vi "3D_send_CCS_command.vi"(0 "CCS IP":string="192.168.000.002", 1 "Intensity 0-255":u8=255, 2 "Light mode":T1(ring), 3 "On/off":bool, 5 "remote port or service name":u16=40001, 7 "Select CCS channel":u16(ring)=2 items=["Chanel 00", "Chanel 01", "Chanel 02"], 9 "Select CCS property":u16(ring)=2 items=["Light Intensity Setting", "Lighting Mode Setting", "ON/OFF Setting"], 11 "error in (no error)":errorcluster) -> (4 "CCS write string":string="@02L0", 15 "error out":errorcluster)   [LabVIEW 2019]
panel:
  out "CCS reply":string
  out "bytes written":i32=9
  out "hex integer string":string="1E"
  out "Write string with checksum":string="@02L01E\r\n"
  # "CCS factory default is 192.168.0.2"
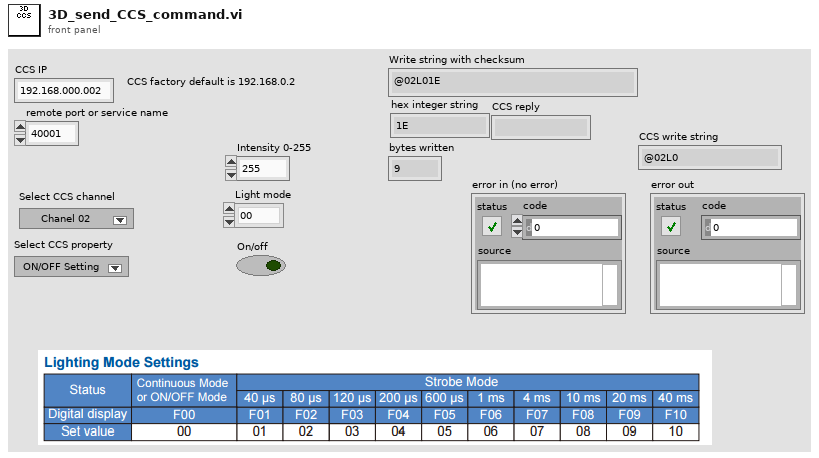
[diagram p1: front panel]
types:
  T1 = enum16{"00", "01", "02", "03", "04", "05", "06", "07", "08", "09", "10"}
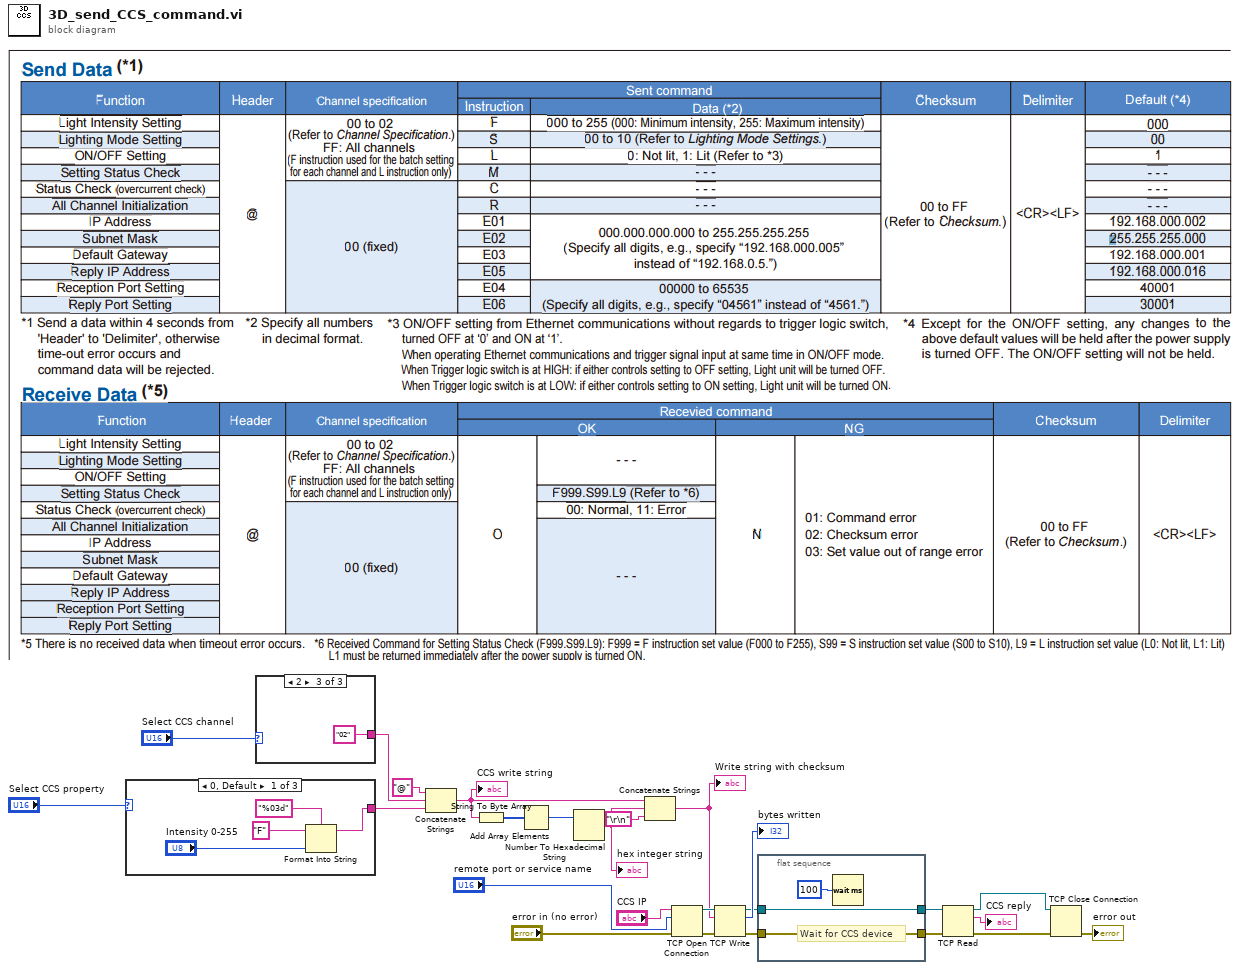
[diagram p0: block diagram]
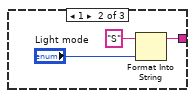
[diagram p2: hidden frame]
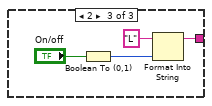
[diagram p3: hidden frame]
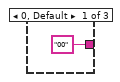
[diagram p4: hidden frame]
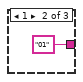
[diagram p5: hidden frame]
diagram:
  n1 = case shown="0, Default" "Select CCS property" {
    tunnel: [w27 w30 w33] -> w21
    frame 0, Default {
      n2 = Format Into String(format string="%03d", initial string="F" ("string"), "Intensity 0-255") -> (resulting string=w27:string)  [unwired: 1 in, 1 out]
    }
    frame 1 {
      n3 = Format Into String(initial string="S" ("string"), "Light mode") -> (resulting string=w30:string)  [unwired: 2 in, 1 out]
    }
    frame 2 {
      n4 = Boolean To (0,1)(Boolean="On/off") -> (0, 1=w34:i16)
      n5 = Format Into String(initial string="L", w34) -> (resulting string=w33:string)  [unwired: 2 in, 1 out]
    }
  }
  n6 = case shown="2" "Select CCS channel" {
    tunnel: ["00" ("string") "01" ("string") "02"] -> w23
    frame 0, Default {
    }
    frame 1 {
    }
    frame 2 {
    }
  }
  n7 = Concatenate Strings("@" ("string"), w23, w21) -> (w1:string)
  "CCS write string" <- w1
  n8 = String To Byte Array(string=w1) -> (unsigned byte array=w20:u8[])
  n9 = Add Array Elements(numeric array=w20) -> (sum=w19:u8)
  n10 = Number To Hexadecimal String(2:w19) -> (0:w18:string)  [unwired: 1 in]
  "hex integer string" <- w18
  n11 = Concatenate Strings(w1, w18, "\r\n") -> (w3:string)
  "Write string with checksum" <- w3
  n12 = TCP Open Connection(address="CCS IP", remote port or service name="remote port or service name", error in (no error)="error in (no error)") -> (connection ID=w16:refnum<k5>, error out=w15:errorcluster)  [unwired: 2 in]
  n13 = TCP Write(connection ID=w16, data in=w3, error in (no error)=w15) -> (connection ID out=w10:refnum<k5>, bytes written=→"bytes written":i32, error out=w9:errorcluster)  [unwired: 1 in]
  n14 = flat-sequence {
    tunnel: w10 -> [w41]
    tunnel: w9 -> [w40]
    tunnel: [w40] -> w8
    tunnel: [w41] -> w5
    frame #0 {
      # "Wait for CCS device"
      n15 = Wait (ms)(milliseconds to wait=u32 100) -> ()  [unwired: 1 out]
    }
  }
  n16 = TCP Read(connection ID=w5, error in (no error)=w8) -> (connection ID out=w4:refnum<k5>, data out=→"CCS reply":string, error out=w7:errorcluster)  [unwired: 3 in]
  n17 = TCP Close Connection(connection ID=w4, error in (no error)=w7) -> (error out=→"error out":errorcluster)  [unwired: 1 in, 1 out]
